vi "dll.midi_disconnect.vi"(8 "error in (no error)":errorcluster, 11 "LabVIEW-MIDI-XPLAT in":refnum<class "midi in.lvclass">) -> (0 "error out":errorcluster, 3 "LabVIEW-MIDI-XPLAT out":refnum<class "midi in.lvclass">)   [LabVIEW 2020, in "MIDIllan.lvlib" / "midi in.lvclass"]
uses:
  midi in.lvclass
  midi in.lvclass/midi in.ctl
  MIDIllan/MIDIllan.lvlib
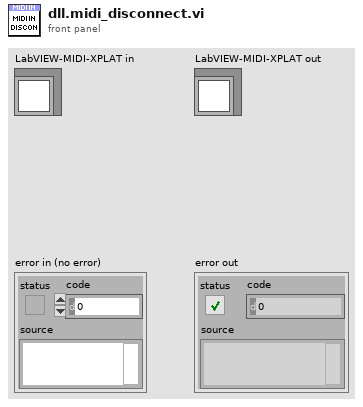
[diagram p1: front panel]
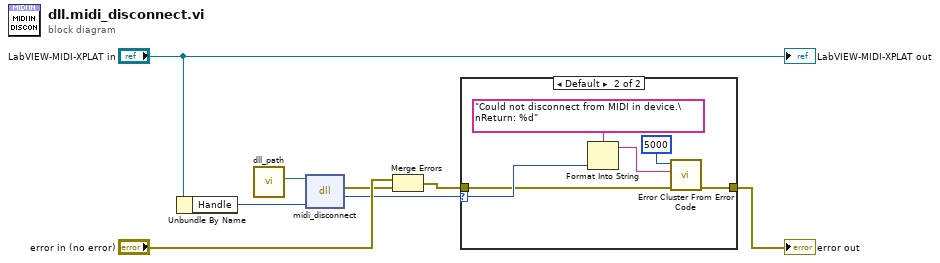
[diagram p0: block diagram]
diagram:
  n1 = Unbundle By Name("LabVIEW-MIDI-XPLAT in") -> ("Handle"=w6:i32)
  n2 = call "dll_path.vi"() -> ("dll"=w7:path)  [unwired: 11 in]
  n3 = dll-call lib="C:/code/LabVIEW-MIDI-XPLAT/dist/TomMIDIllan_*.*" fn="midi_disconnect"(path in=w7, "handle"=w6) -> (error out=w4:errorcluster, "return"=w2:i32)  [unwired: 3 in, 1 out]
  n4 = Merge Errors("error in (no error)", w4) -> (w3:errorcluster)
  n5 = case shown="Default" w2 {
    selector: w2 -> [_ w12]
    tunnel: w3 -> [w9 w11]
    tunnel: [w9 w10] -> w1
    frame 0.. {
    }
    frame Default {
      n6 = Format Into String(format string="Could not disconnect from MIDI in device.\nReturn: %d", w12) -> (resulting string=w13:string)  [unwired: 2 in, 1 out]
      n7 = call <vilib>:"Error Cluster From Error Code.vi"("error in (no error)"=w11, "error message (\"\")"=w13, "error code (0)"=5000) -> ("error out"=w10:errorcluster)  [unwired: 6 in]
    }
  }
  "error out" <- w1
  "LabVIEW-MIDI-XPLAT out" <- "LabVIEW-MIDI-XPLAT in"
